vi "main_SK.vi"() -> ()   [LabVIEW 2017]
panel:
  in  "ActiveSensor":u16(ring) items=["Ultrasonic", "Thermocouple / Heater", "Humidity", "Flow Rate", "Load Cell", "Solenoid Valve", "Pressure Sensor / Compressor", ""]
  in  "Exit":bool
  out "NI1":tag caption="NI device"
  in  "ActiveSensorTab":T1(tab) caption="Active sensor/actuator window"
  out "Ultrasonic Output":bool
  out "Ultrasonic Chart":dbl(graph)
  out "T3":dbl
  out "T2":dbl
  out "T1":dbl
  in  "Heater ON/OFF":bool
  out "Heater LED":bool
  out "Thermocouples Chart":T2(graph)
  out "Humidity":dbl
  out "Humidity Chart":dbl(graph)
  out "Flow rate":dbl
  out "Flowrate Chart":dbl(graph)
  out "Load":dbl
  out "Load Chart":dbl(graph)
  out "Solenoid Valve":bool
  in  "Valve ON/OFF":bool
  out "Compresssor LED":bool
  in  "Compressor ON/OFF":bool
  out "Pressure reading":dbl
  out "Pressure Chart":cluster{"Scalar":dbl, i16}(graph)
  # "Sensor Kit"
  # "Choose Kit :"
  # "1"
  # "0"
  # "Temperatrure readings"
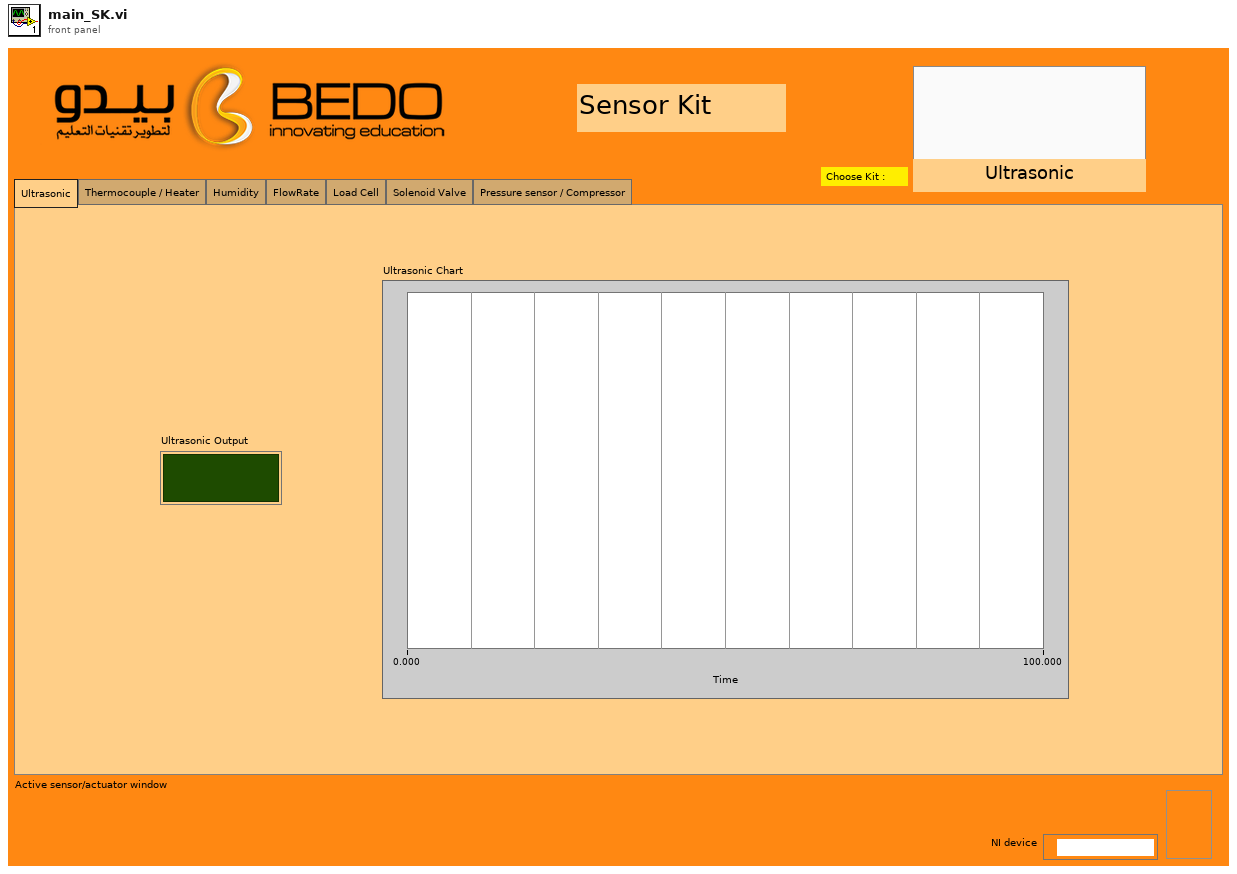
[diagram p1: front panel]
types:
  T1 = enum32{"Ultrasonic", "Thermocouple / Heater", "Humidity", "FlowRate", "Load Cell", "Solenoid Valve", "Pressure sensor / Compressor"}
  T2 = cluster{"Scalar":dbl, "Scalar":dbl, "Scalar":dbl, i16}
  T3 = enum32{"Invalid", "Standard", "Closed", "Hidden", "Minimized", "Maximized"}
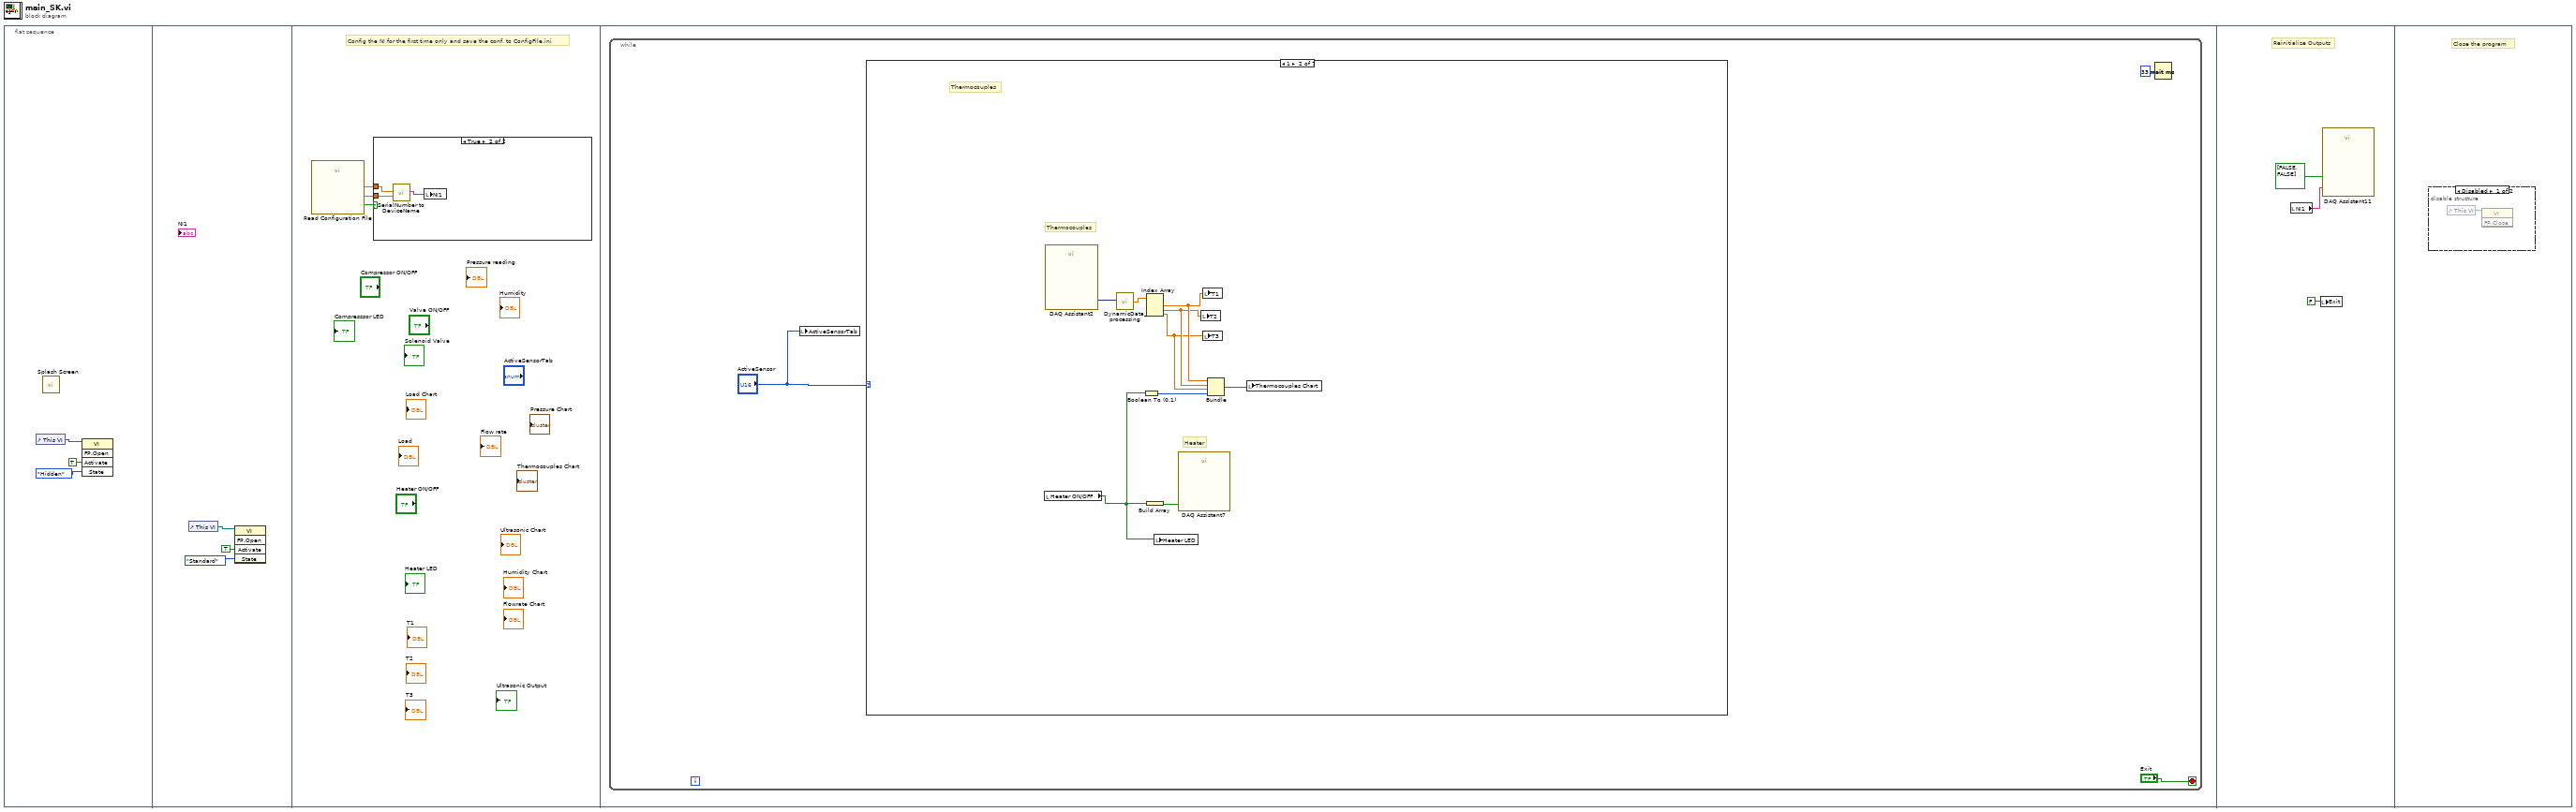
[diagram p0: block diagram]
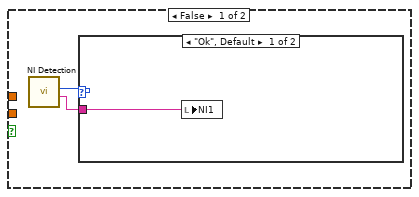
[diagram p2: hidden frame]
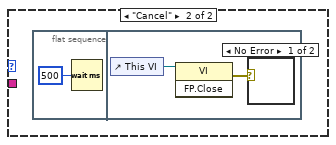
[diagram p3: hidden frame]
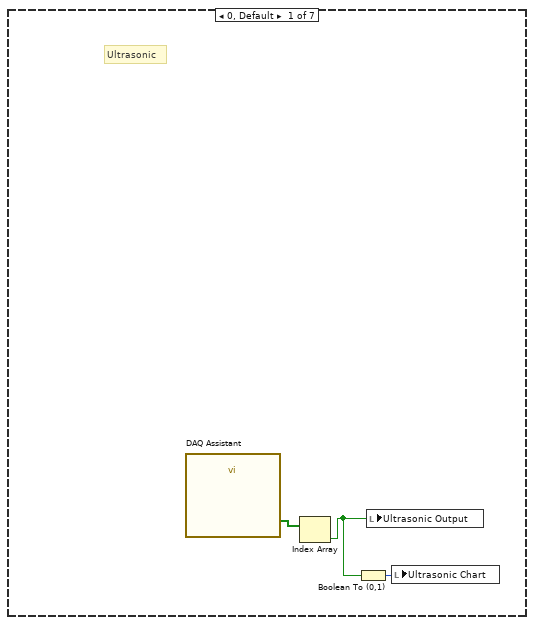
[diagram p5: hidden frame]
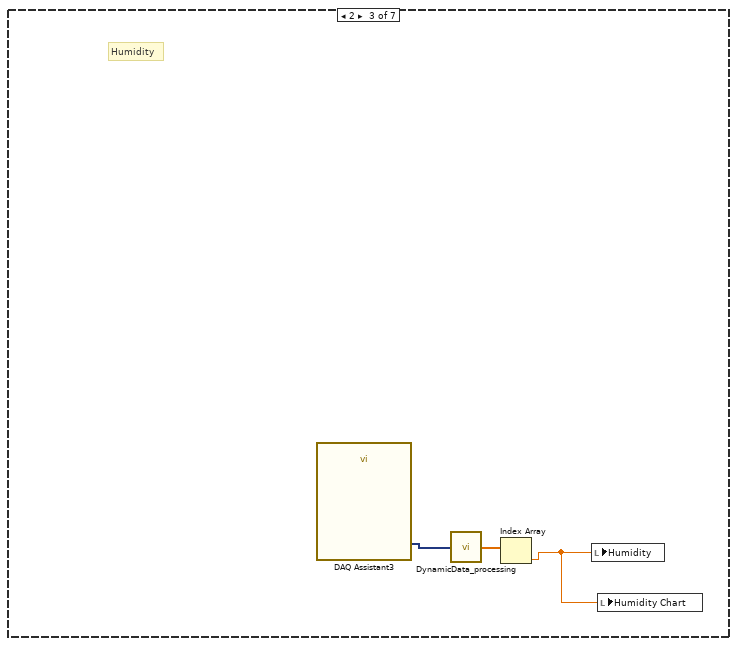
[diagram p6: hidden frame]
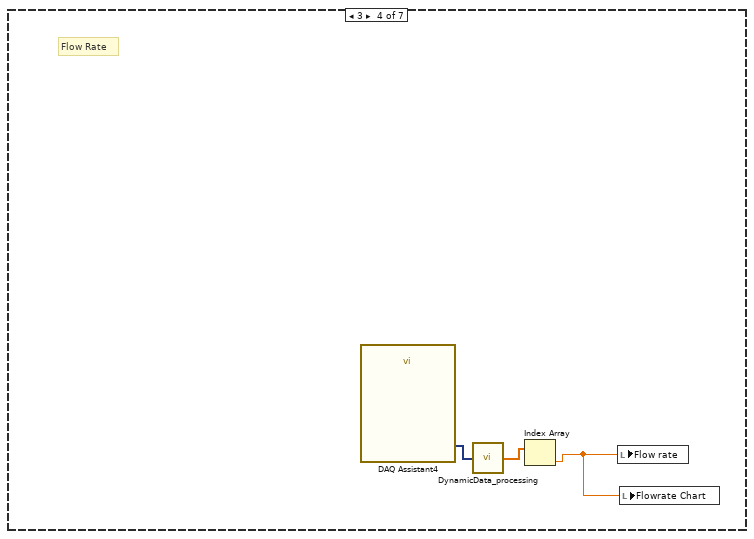
[diagram p7: hidden frame]
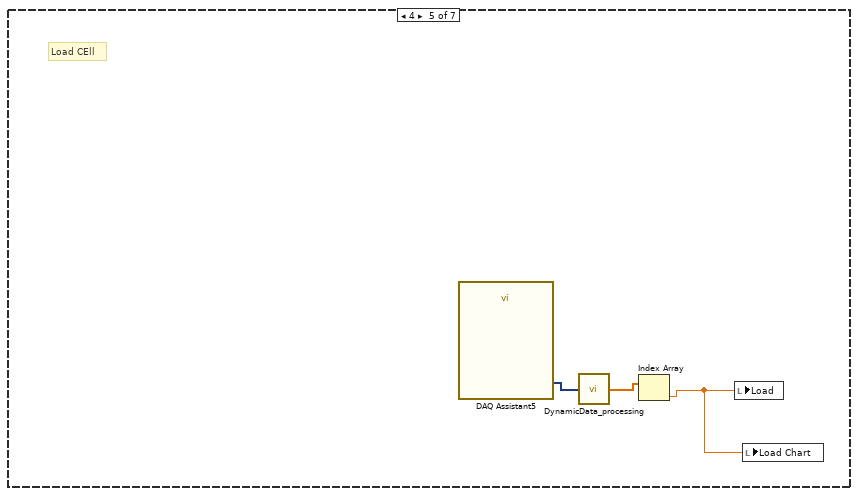
[diagram p8: hidden frame]
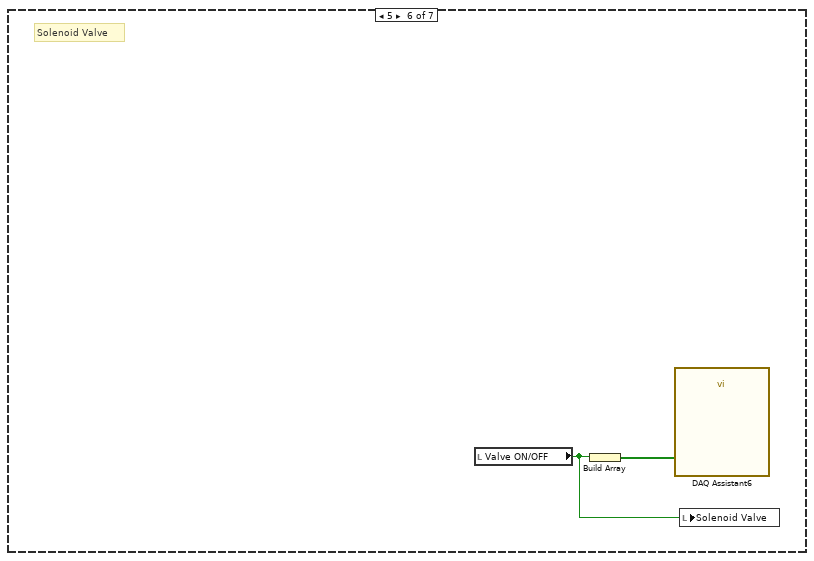
[diagram p9: hidden frame]
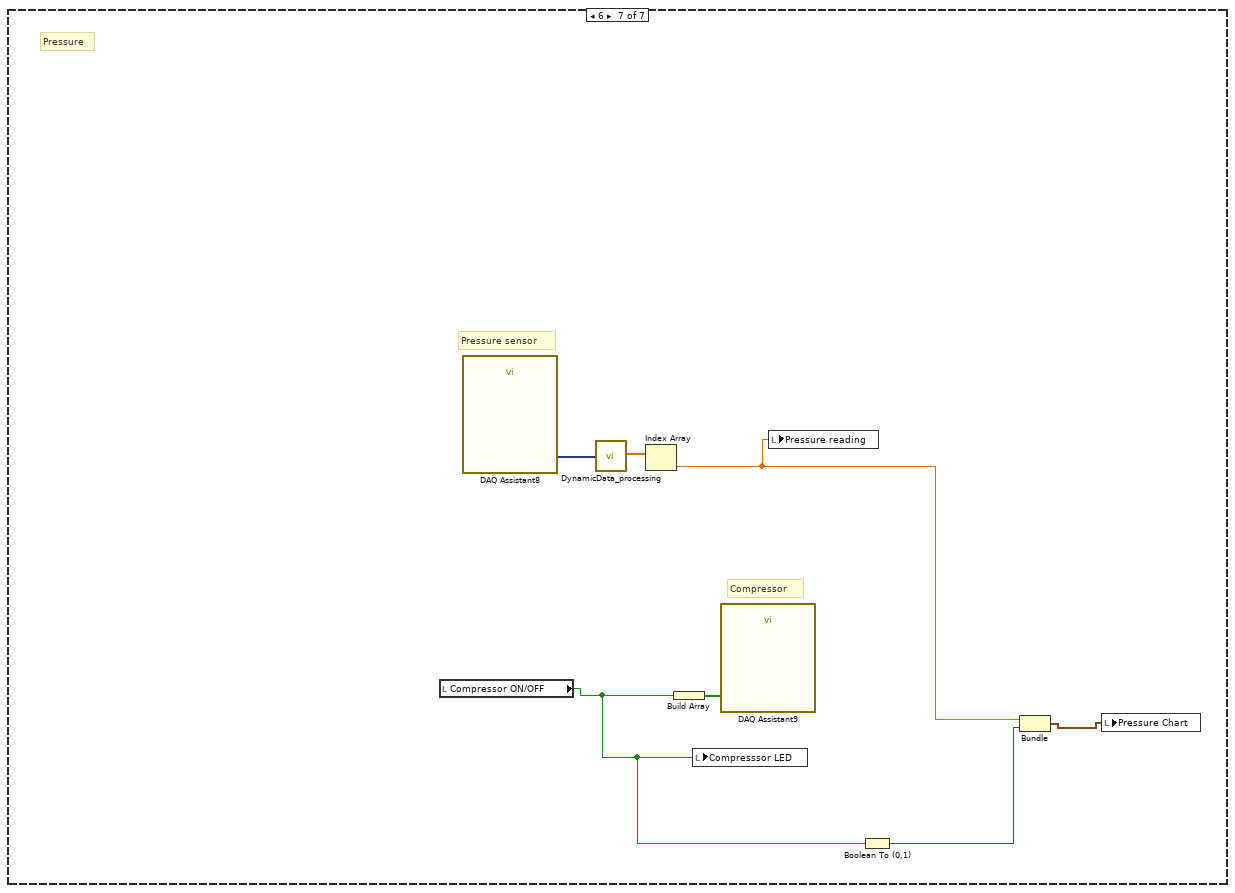
[diagram p10: hidden frame]
diagram:
  n1 = flat-sequence {
    frame #0 {
      n2 = control-ref of="This VI"() -> (w3:refnum<vi>)
      n3 = call "Splash Screen.vi"() -> ()  [unwired: 11 in, 1 out]
      n4 = invoke class="VI" method="FP.Open"(reference=w3, "Activate"=TRUE ("Activate?"), "State"=T3."Hidden") -> ()  [unwired: 2 in, 5 out]
    }
    frame #1 {
      n5 = control-ref of="This VI"() -> (w4:refnum<vi>)
      n6 = invoke class="VI" method="FP.Open"(reference=w4, "Activate"=TRUE ("Activate?"), "State"=T3."Standard") -> ()  [unwired: 2 in, 5 out]
    }
    frame #2 {
      # "Config the NI for the first time only and save the conf. to ConfigFile.ini"
      n7 = call "Read Configuration File.vi"() -> ("Serial Numbers Found"=w7:bool, "NI1"=w8:dbl, "NI2"=w9:dbl)  [unwired: 13 in]
      n8 = case shown="True" w7 {
        tunnel: w8 -> [_ w18]
        tunnel: w9 -> [_ w17]
        frame False {
          n9 = call "NI Detection.vi"() -> ("NI 1"=w10:tag, "Ok/Cancel"=w11:enum16{"Ok", "Cancel"})  [unwired: 8 in, 1 out]
          n10 = case shown="\"Ok\", Default" w11 {
            tunnel: w10 -> [w12 _]
            frame "Ok", Default {
              n11 = local write "NI1"(w12) -> ()
            }
            frame "Cancel" {
              n12 = flat-sequence {
                frame #0 {
                  n13 = Wait (ms)(milliseconds to wait=u32 500) -> ()  [unwired: 1 out]
                }
                frame #1 {
                  n14 = control-ref of="This VI"() -> (w15:refnum<vi>)
                  n15 = invoke class="VI" method="FP.Close"(reference=w15) -> (error out=w14:errorcluster)  [unwired: 2 in, 2 out]
                  n16 = case shown="No Error" w14 {
                    frame No Error {
                    }
                    frame Error {
                    }
                  }
                }
              }
            }
          }
        }
        frame True {
          n17 = call "SerialNumber to DeviceName.vi"("NI2 Serial Number"=w17, "NI1 Serial Number"=w18) -> ("NI1 Device Name"=w16:tag)  [unwired: 8 in, 1 out]
          n18 = local write "NI1"(w16) -> ()
        }
      }
    }
    frame #3 {
      n19 = while {
        stop <- "Exit" stop-if-true
        n20 = local write "ActiveSensorTab"("ActiveSensor") -> ()
        n21 = case shown="1" "ActiveSensor" {
          frame 0, Default {
            # "Ultrasonic"
            n22 = call "DAQ Assistant"() -> ("data"=w24:bool[])  [unwired: 17 in, 2 out]
            n23 = Index Array(array=w24) -> (element=w23:bool)  [unwired: 1 in]
            n24 = Boolean To (0,1)(Boolean=w23) -> (0, 1=w22:i16)
            n25 = local write "Ultrasonic Output"(w23) -> ()
            n26 = local write "Ultrasonic Chart"(w22) -> ()
          }
          frame 1 {
            # "Heater"
            # "Thermocouples"
            # "Thermocouples"
            n27 = local read "Heater ON/OFF"() -> (w27:bool)
            n28 = call "DAQ Assistant2"() -> ("data"=w33:dynamicdata)  [unwired: 17 in, 2 out]
            n29 = call "DynamicData_processing.vi"("data"=w33) -> ("DATA"=w32:dbl[])
            n30 = Boolean To (0,1)(Boolean=w27) -> (0, 1=w26:i16)
            n31 = Index Array(array=w32) -> (element #1=w31:dbl, element #2=w30:dbl, element #3=w29:dbl)  [unwired: 3 in]
            n32 = Build Array(w27) -> (w28:bool[])
            n33 = local write "Heater LED"(w27) -> ()
            n34 = call "DAQ Assistant7"("data"=w28) -> ()  [unwired: 17 in, 2 out]
            n35 = local write "T2"(w30) -> ()
            n36 = local write "T1"(w31) -> ()
            n37 = local write "T3"(w29) -> ()
            n38 = Bundle("Scalar"=w31, "Scalar"=w30, "Scalar"=w29, w26) -> (w25:T2)  [unwired: 1 in]
            n39 = local write "Thermocouples Chart"(w25) -> ()
          }
          frame 2 {
            # "Humidity"
            n40 = call "DAQ Assistant3"() -> ("data"=w36:dynamicdata)  [unwired: 17 in, 2 out]
            n41 = call "DynamicData_processing.vi"("data"=w36) -> ("DATA"=w35:dbl[])
            n42 = Index Array(array=w35) -> (element=w34:dbl)  [unwired: 1 in]
            n43 = local write "Humidity"(w34) -> ()
            n44 = local write "Humidity Chart"(w34) -> ()
          }
          frame 3 {
            # "Flow Rate"
            n45 = call "DAQ Assistant4"() -> ("data"=w39:dynamicdata)  [unwired: 17 in, 2 out]
            n46 = call "DynamicData_processing.vi"("data"=w39) -> ("DATA"=w38:dbl[])
            n47 = Index Array(array=w38) -> (element=w37:dbl)  [unwired: 1 in]
            n48 = local write "Flow rate"(w37) -> ()
            n49 = local write "Flowrate Chart"(w37) -> ()
          }
          frame 4 {
            # "Load CEll"
            n50 = call "DAQ Assistant5"() -> ("data"=w42:dynamicdata)  [unwired: 17 in, 2 out]
            n51 = call "DynamicData_processing.vi"("data"=w42) -> ("DATA"=w41:dbl[])
            n52 = Index Array(array=w41) -> (element=w40:dbl)  [unwired: 1 in]
            n53 = local write "Load"(w40) -> ()
            n54 = local write "Load Chart"(w40) -> ()
          }
          frame 5 {
            # "Solenoid Valve"
            n55 = local read "Valve ON/OFF"() -> (w43:bool)
            n56 = Build Array(w43) -> (w44:bool[])
            n57 = call "DAQ Assistant6"("data"=w44) -> ()  [unwired: 17 in, 2 out]
            n58 = local write "Solenoid Valve"(w43) -> ()
          }
          frame 6 {
            # "Compressor"
            # "Pressure sensor"
            # "Pressure"
            n59 = local read "Compressor ON/OFF"() -> (w46:bool)
            n60 = call "DAQ Assistant8"() -> ("data"=w51:dynamicdata)  [unwired: 17 in, 2 out]
            n61 = call "DynamicData_processing.vi"("data"=w51) -> ("DATA"=w50:dbl[])
            n62 = Index Array(array=w50) -> (element=w48:dbl)  [unwired: 1 in]
            n63 = Build Array(w46) -> (w49:bool[])
            n64 = local write "Compresssor LED"(w46) -> ()
            n65 = call "DAQ Assistant9"("data"=w49) -> ()  [unwired: 17 in, 2 out]
            n66 = local write "Pressure reading"(w48) -> ()
            n67 = Boolean To (0,1)(Boolean=w46) -> (0, 1=w47:i16)
            n68 = Bundle("Scalar"=w48, w47) -> (w45:cluster{"Scalar":dbl, i16})  [unwired: 1 in]
            n69 = local write "Pressure Chart"(w45) -> ()
          }
        }
        n70 = Wait (ms)(milliseconds to wait=u32 33) -> ()  [unwired: 1 out]
      }
    }
    frame #4 {
      # "Reinitialize Outputs"
      n71 = local read "NI1"() -> (w53:tag)
      n72 = local write "Exit"(FALSE ("Exit")) -> ()
      n73 = call "DAQ Assistant11"("data"=bool[] [FALSE, FALSE], "device name"=w53) -> ()  [unwired: 16 in, 2 out]
    }
    frame #5 {
      # "Close the program"
      n74 = disable-structure shown="Disabled" {
        frame Disabled {
          n75 = control-ref of="This VI"() -> (w55:refnum<vi>)
          n76 = invoke class="VI" method="FP.Close"(reference=w55) -> ()  [unwired: 2 in, 3 out]
        }
        frame Enabled {
        }
      }
    }
  }
